vi "StepRealtime_IP5.vi"() -> ()   [LabVIEW 2011]
doc: "This VI was generated automatically using the FPGA Wizard. You can modify the VI normally."
uses:
  <vilib>/Platform/TimedLoop/XDataNode/timing_clust.ctl
  <vilib>/Platform/TimedLoop/XDataNode/nitl_modes.ctl
  <vilib>/Platform/TimedLoop/XDataNode/wakeup.ctl
  <vilib>/FPGAPlugInAG/sbRIO-9632/niLvFpga_Open_sbRIO-9632.vi
  <vilib>/rvi/interface/common/dynamic/niFpgaDynamicAddResources.vi
  <vilib>/FPGAPlugInAG/Dynamic/niLvFpga_Reset_Dynamic.vi
  <vilib>/FPGAPlugInAG/Dynamic/niLvFpga_Download_Dynamic.vi
  <vilib>/FPGAPlugInAG/Dynamic/niLvFpga_Run_Dynamic.vi
  <vilib>/Utility/error.llb/Error Cluster From Error Code.vi
  <vilib>/rvi/errors/niLvFpgaAdjustHostInterfaceError.vi
  <vilib>/FPGAPlugInAG/Dynamic/niLvFpga_Close_Dynamic.vi
  <vilib>/rvi/interface/nirviOpenFPGA/nirviOpenFPGA.xnode
  FPGA Bitfiles/PPDControlLab3_FPGA_IP5.lvbitx
  <vilib>/rvi/interface/nirviMethod/nirviMethod.xnode
  <vilib>/Platform/TimedLoop/XDataNode/XDataNode.xnode
  <vilib>/rvi/interface/nirviReadWriteControl/nirviReadWriteControl.xnode
  <vilib>/rvi/interface/nirviCloseFPGA/nirviCloseFPGA.xnode
  SysIDRealtime.lvlib
  <vilib>/rvi/interface/Simulation/niFpgaSimulationCallBeginRW.vi
  <vilib>/Platform/TimedLoop/XDataNode/XDNodeRunTimeDep.lvlib
  NiFpgaLv.dll
panel:
  out "Ratio":fxp<+/-,32,7>
  in  "Gain":fxp<+/-,32,7>=0.006999999284744263
  in  "Radio Buttons":enum32{"Radio Selection 1", "Radio Selection 2"}(radio)
  in  "OK Button":bool
  out "Step Response":dynamicdata(graph)=[{"t0"=timestamp(0 s since 1904-01-01), "dt"=1.0, "Y"=array[2048 elements]}, {"t0"=timestamp(0 s since 1904-01-01), "dt"=1.0, "Y"=array[2048 elements]}, {"t0"=timestamp(0 s since 1904-01-01), "dt"=1.0, "Y"=array[2048 elements]}]
  in  "samples":i32=2048
  in  "Reference":i32=100000
  in  "Quad Reset":bool=TRUE
  in  "DGain":fxp<+/-,32,7>
  in  "PGain":fxp<+/-,32,7>
  out "Amp In":dbl[](graph)
  out "Amp Cpmmand":fxp<+/-,20,5>
  out "Iteration Duration":i64
  out "Position":i32[](graph)
  in  "Control Rate (ticks)":u32=10000
  in  "Period (us)":i64=1000
  out "Finished Late? [i-1]":bool
  out "quad saved (Port0/DIO0,Port0/DIO1)":cluster{"Position":i32, "Index Count":u16}
  out "quad pos (Port0/DIO0,Port0/DIO1)":i32
  out "Late? Latched":bool
  in  "Local Stop 0":bool
  in  "Start 0":bool
  in  "Loop Rate (Hz)":dbl=100000.0
  out "Calculated Rate (Hz)":dbl
  out "error out":errorcluster
  in  "Global Stop":bool
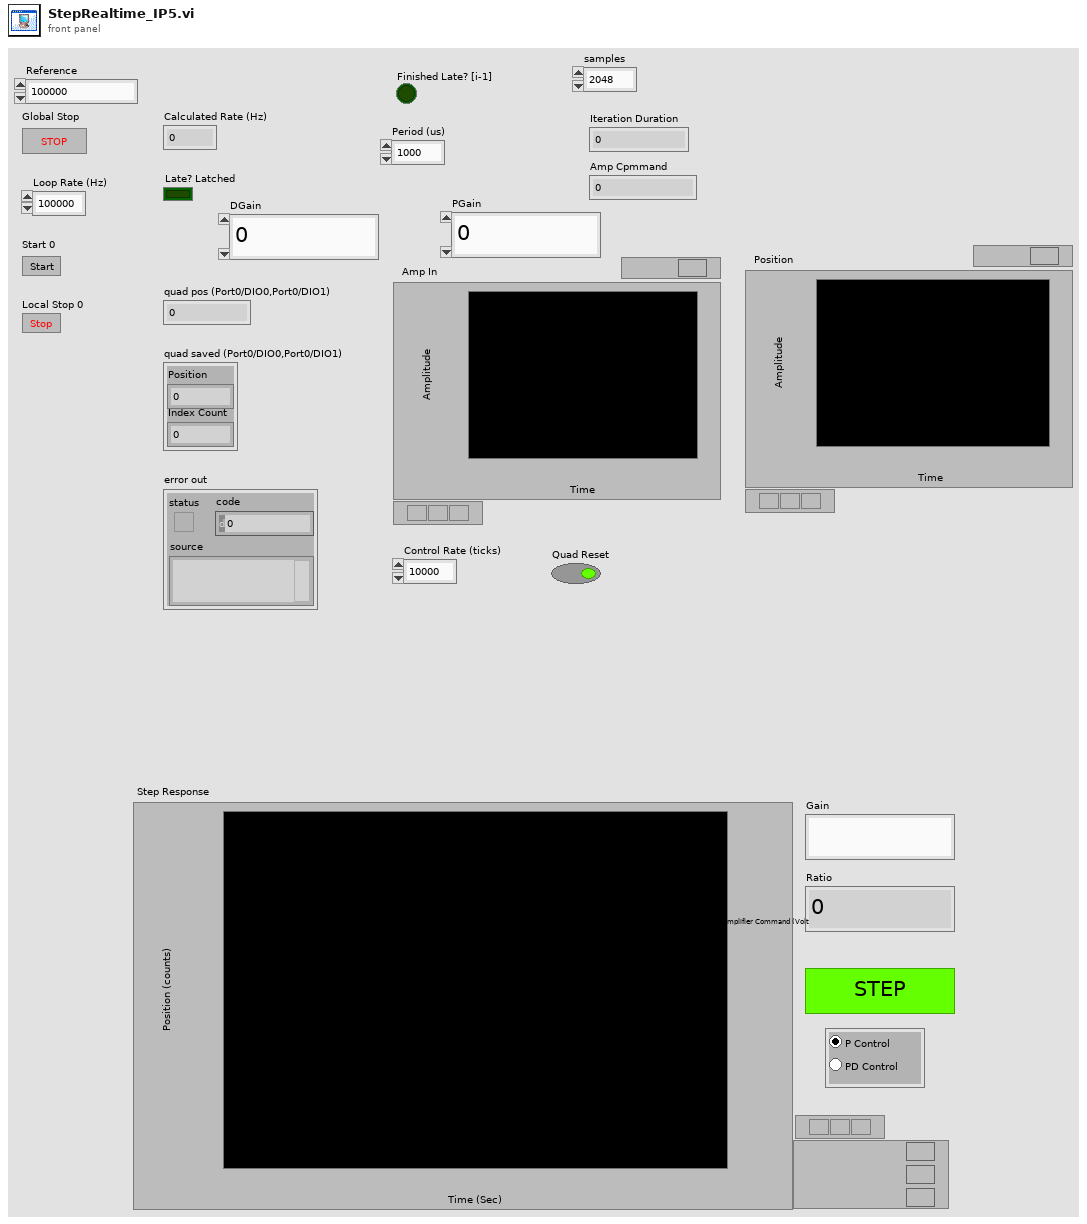
[diagram p1: front panel]
types:
  T1 = typedef "XDNodeRunTimeDep.lvlib/timing_clust.ctl" = cluster{"Expected End [f-1]":u64, "Actual End [f-1]":u64, "Finished Late? [f-1]":bool, "Expected End [i-1]":u64, "Actual End [i-1]":u64, "Finished Late? [i-1]":bool, "Expected Start [i]":u64, "Actual Start [i]":u64, "Expected Start [f]":u64, "Actual Start [f]":u64, "Source Name":string, "Structure Name":string, "Period":i64, "Deadline":i64, "Offset":i64, "Start":i64, "Priority":i32, "Timeout":i32, "Mode":T2, "Wakeup Reason":T3, "Error":errorcluster, "Source Type":string, "Secondary Source Type":string, "Global End Time":u64, "Global Start Time":u64, "Frame Duration":u64, "Iteration Duration":u64, "Assigned CPU":i32, "I/O Scan Engine Mode":u32}
  T2 = typedef "XDNodeRunTimeDep.lvlib/nitl_modes.ctl" = enum32{"No Change", "Process missed periods, maintain original phase", "Discard missed periods, maintain original phase", "Process missed periods, ignore original phase", "Discard missed periods, ignore original phase"}
  T3 = typedef "XDNodeRunTimeDep.lvlib/wakeup.ctl" = enum32{"Normal", "Aborted", "Asynchronous wakeup", "Timing source error", "Timed loop error", "Timeout"}
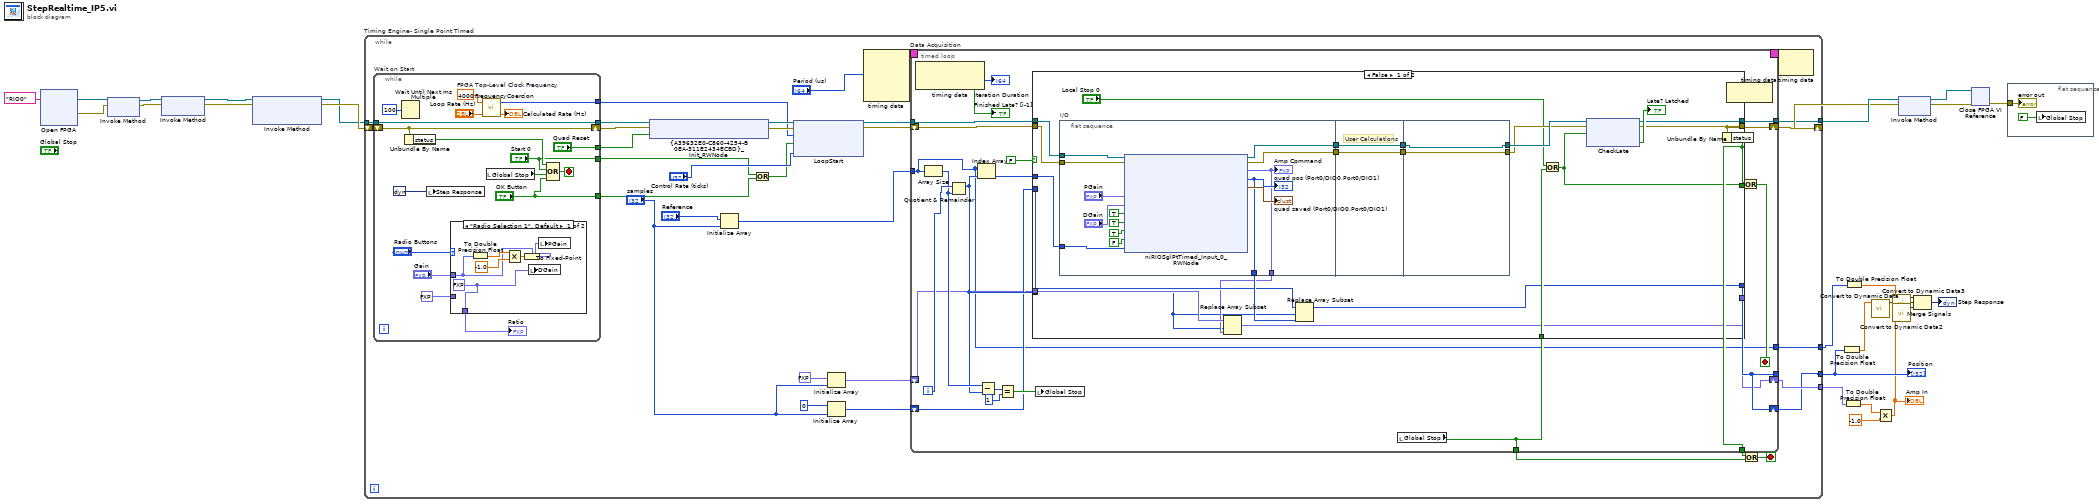
[diagram p0: block diagram]
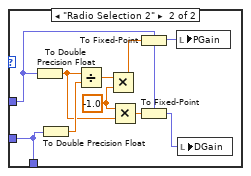
[diagram p3: hidden frame]
diagram:
  n1 = xnode ("Open FPGA")("resource name"=tag "RIO0") -> ("FPGA VI Reference Out"=w24:refnum<k20>, "error out"=w25:errorcluster)  [unwired: 1 in]
  n2 = xnode ("Invoke Method")("FPGA VI Reference In"=w24, "error in"=w25) -> ("FPGA VI Reference Out"=w4:refnum<k20>, "error out"=w3:errorcluster)
  n3 = xnode ("Invoke Method")("FPGA VI Reference In"=w4, "error in"=w3) -> ("FPGA VI Reference Out"=w1:refnum<k20>, "error out"=w2:errorcluster)
  n4 = xnode ("Invoke Method")("FPGA VI Reference In"=w1, "error in"=w2) -> ("FPGA VI Reference Out"=w12:refnum<k20>, "error out"=w26:errorcluster)  [unwired: 1 in]
  n5 = while "Timing Engine- Single Point Timed" {
    tunnel: w12 -> [w55]
    shift-right: [w54] -> w10
    shift-left: w26 -> [w58]
    tunnel: [w36] -> w18
    tunnel: [w37] -> w22
    tunnel: [w31] -> w16
    tunnel: [w27] -> w11
    stop <- w49 stop-if-true
    n6 = while "Wait on Start" {
      tunnel: w55 -> [w149]
      tunnel: [w149] -> w53
      tunnel: [w141] -> w46
      tunnel: ["Start 0"] -> w30
      shift-right: [w143] -> w52
      shift-left: w58 -> [w143]
      tunnel: ["Quad Reset"] -> w35
      tunnel: ["OK Button"] -> w29
      stop <- w150 stop-if-true
      w144 = 40000000.0  # FPGA Top-Level Clock Frequency
      n7 = Wait Until Next ms Multiple(millisecond multiple=u32 100) -> ()  [unwired: 1 out]
      n8 = Unbundle By Name(w143) -> ("status"=w142:bool)
      n9 = local write "Step Response"(dynamicdata [] ("Step Response")) -> ()
      n10 = case shown="\"Radio Selection 1\", Default" "Radio Buttons" {
        tunnel: "Gain" -> [w152 w158]
        tunnel: fxp<+/-,32,7> 40.0 ("Ratio") -> [_ w163]
        tunnel: [w156 w163] -> w134
        frame "Radio Selection 1", Default {
          w156 = fxp<+/-,32,7> 0.0 ("DGain")
          n11 = To Double Precision Float(number=w152) -> (double precision float=w155:dbl)
          n12 = Multiply(x=w155, y=-1.0) -> (x*y=w153:dbl)
          n13 = To Fixed-Point(fixed-point type=w152, number=w153) -> (fixed-point=w151:fxp<+/-,32,7>)
          n14 = local write "DGain"(w156) -> ()
          n15 = local write "PGain"(w151) -> ()
        }
        frame "Radio Selection 2" {
          w161 = -1.0 ("y")
          n16 = To Double Precision Float(number=w158) -> (double precision float=w160:dbl)
          n17 = To Double Precision Float(number=w163) -> (double precision float=w166:dbl)
          n18 = Divide(x=w160, y=w166) -> (x/y=w165:dbl)
          n19 = Multiply(x=w165, y=w161) -> (x*y=w162:dbl)
          n20 = Multiply(x=w161, y=w160) -> (x*y=w159:dbl)
          n21 = To Fixed-Point(fixed-point type=w158, number=w162) -> (fixed-point=w164:fxp<+/-,32,7>)
          n22 = To Fixed-Point(fixed-point type=w158, number=w159) -> (fixed-point=w157:fxp<+/-,32,7>)
          n23 = local write "PGain"(w164) -> ()
          n24 = local write "DGain"(w157) -> ()
        }
      }
      "Ratio" <- w134
      n25 = call "FrequencyCoercion.vi"("Loop Rate (Hz)"="Loop Rate (Hz)", "FPGA Top-Level Clock Frequency"=w144) -> ("Actual Rate (Hz)"=→"Calculated Rate (Hz)":dbl, "FPGA Ticks"=w141:u32)  [unwired: 2 in]
      n26 = local read "Global Stop"() -> (w147:bool)
      n27 = Compound Arithmetic op=OR(w142, "Start 0", w147, "OK Button") -> (w150:bool)
    }
    n28 = xnode ("{A39632E0-C860-4254-B0EA-311E2434ECBD}_Init_RWNode")("FPGA VI Reference In"=w53, "error in"=w52, "quad reset (Port0/DIO0,Port0/DIO1)"=w35) -> ("FPGA VI Reference Out"=w47:refnum<k20>, "error out"=w51:errorcluster)
    n29 = Initialize Array("Reference", "samples") -> (w32:i32[])
    n30 = Or(x=w30, y=w29) -> (x .or. y?=w28:bool)
    n31 = xnode ("LoopStart")("FPGA VI Reference In"=w47, "error in"=w51, "Loop Rate (Ticks)"=w46, "Start 0"=w28, "Control Rate (ticks)"="Control Rate (ticks)") -> ("FPGA VI Reference Out"=w57:refnum<k20>, "error out"=w56:errorcluster)
    n32 = Initialize Array(0 ("quad pos (Port0/DIO0,Port0/DIO1)"), "samples") -> (w40:i32[])
    n33 = Initialize Array(fxp<+/-,20,5> 0.0 ("Amp Cpmmand"), "samples") -> (w38:fxp<+/-,20,5>[])
    n34 = node-c288("Period (us)") -> (w45:T1)  [unwired: 3 in]
    n35 = timed-loop "Data Acquisition" {
      tunnel: w57 -> [w76]
      tunnel: [w78] -> w50
      tunnel: [w77] -> w48
      shift-right: [w81] -> w54
      shift-left: w56 -> [w75]
      timing: w45 -> [_]
      timing-out: [_] -> w44
      tunnel: w32 -> [w60]
      tunnel: [w62] -> _
      shift-right: [w61] -> w37
      shift-left: w38 -> [w63]
      shift-right: [w62] -> w36
      shift-left: w40 -> [w65]
      tunnel: [w60] -> w31
      tunnel: [w59] -> w27
      i -> [w72]
      stop <- w79 stop-if-true
      n36 = node-c288() -> (→"Finished Late? [i-1]":bool, →"Iteration Duration":i64)  [unwired: 1 in]
      n37 = Array Size(array=w60) -> (size(s)=w70:i32)
      n38 = Quotient & Remainder(x=w72, y=w70) -> (x-y*floor(x/y)=w66:i32)  [unwired: 1 out]
      n39 = Index Array(array=w60, index=w66) -> (element=w71:i32)
      n40 = Subtract(x=w70, y=w66) -> (x-y=w69:i32)
      n41 = Equal?(x=w69, y=1) -> (x = y?=w67:bool)
      n42 = local write "Global Stop"(w67) -> ()
      n43 = local read "Global Stop"() -> (w78:bool)
      n44 = case "Timeout" shown="False" FALSE {
        tunnel: w76 -> [w102 w126]
        tunnel: w75 -> [w101 w128]
        tunnel: [w95 w128] -> w81
        tunnel: [w97 w127] -> w80
        tunnel: w78 -> [w98 w127]
        tunnel: w71 -> [w87 _]
        tunnel: w66 -> [w89 _]
        tunnel: w65 -> [w93 _]
        tunnel: [w92 _] -> w62
        tunnel: w63 -> [w91 _]
        tunnel: [w88 _] -> w61
        tunnel: [w86 w126] -> w59
        frame False {
          n45 = flat-sequence "I/O" {
            tunnel: w102 -> [w119]
            tunnel: w101 -> [w121]
            tunnel: [w120] -> w107
            tunnel: [w118] -> w104
            tunnel: [w116] -> w94
            tunnel: [w115] -> w90
            tunnel: w87 -> [w108]
            tunnel: [w123] -> w106
            tunnel: w107 -> [w122]
            tunnel: w104 -> [w123]
            tunnel: [w122] -> w105
            tunnel: [w124] -> w100
            tunnel: [w125] -> w103
            tunnel: w106 -> [w125]
            tunnel: w105 -> [w124]
            frame #0 {
              n46 = xnode ("niRIOSglPtTimed_Input_0_RWNode")("FPGA VI Reference In"=w119, "error in"=w121, "PGain"="PGain", "DGain"="DGain", "Amp Enable"=TRUE, "Amp Reset"=TRUE, "Brake"=TRUE, "quad reset (Port0/DIO0,Port0/DIO1)"=FALSE, "Reference"=w108) -> ("FPGA VI Reference Out"=w118:refnum<k20>, "error out"=w120:errorcluster, "Amp Cpmmand"=w115:fxp<+/-,20,5>, "_quad pos (Port0/DIO0,Port0/DIO1)"=w116:i32, "quad saved (Port0/DIO0,Port0/DIO1)"=→"quad saved (Port0/DIO0,Port0/DIO1)":cluster{"Position":i32, "Index Count":u16})
              "quad pos (Port0/DIO0,Port0/DIO1)" <- w116
              "Amp Cpmmand" <- w115
            }
            frame #1 {
              # "User Calculations"
            }
            frame #2 {
            }
          }
          n47 = Replace Array Subset(array=w91, new element=w90, index=w89) -> (w88:fxp<+/-,20,5>[])
          n48 = Replace Array Subset(array=w93, new element=w94, index=w89) -> (w92:i32[])
          n49 = Or(x="Local Stop 0", y=w98) -> (x .or. y?=w97:bool)
          n50 = xnode ("CheckLate")("FPGA VI Reference In"=w103, "error in"=w100, "Local Stop 0"=w97) -> ("FPGA VI Reference Out"=w86:refnum<k20>, "error out"=w95:errorcluster, "Late? Latched"=→"Late? Latched":bool)
        }
        frame True {
          # "Timeout waiting for an interrupt. This case checks the state of the global stop.\nIf global stop is not set, then loop around to wait for an interrupt again."
        }
      }
      n51 = Unbundle By Name(w81) -> ("status"=w77:bool)
      n52 = node-c288() -> ()  [unwired: 1 in, 1 out]
      n53 = Or(x=w77, y=w80) -> (x .or. y?=w79:bool)
    }
    n54 = Or(x=w48, y=w50) -> (x .or. y?=w49:bool)
    n55 = node-c288(w44) -> ()  [unwired: 1 out]
  }
  "Position" <- w18
  n56 = To Double Precision Float(number=w18) -> (double precision float=w17:dbl[])
  n57 = To Double Precision Float(number=w22) -> (double precision float=w6:dbl[])
  n58 = To Double Precision Float(number=w16) -> (double precision float=w15:dbl[])
  n59 = call "Convert to Dynamic Data"("Array"=w17) -> ("Dynamic Data Type"=w20:dynamicdata)  [unwired: 3 in]
  n60 = Multiply(x=w6, y=-1.0) -> (x*y=w5:dbl[])
  "Amp In" <- w5
  n61 = call "Convert to Dynamic Data3"("Array"=w15) -> ("Dynamic Data Type"=w14:dynamicdata)  [unwired: 3 in]
  n62 = call "Convert to Dynamic Data2"("Array"=w5) -> ("Dynamic Data Type"=w19:dynamicdata)  [unwired: 3 in]
  n63 = xnode "Invoke Method"("FPGA VI Reference In"=w11, "error in"=w10) -> ("FPGA VI Reference Out"=w9:refnum<k20>, "error out"=w8:errorcluster)
  n64 = Merge Signals(w14, w20, w19) -> (→"Step Response":dynamicdata)
  n65 = xnode ("Close FPGA VI Reference")("FPGA VI Reference In"=w9, "error in"=w8) -> ("error out"=w23:errorcluster)
  n66 = flat-sequence {
    tunnel: w23 -> [w168]
    frame #0 {
      n67 = local write "Global Stop"(FALSE ("Global Stop")) -> ()
      "error out" <- w168
    }
  }
